vi "Merge_Files.vi"(8 "error in (no error)":errorcluster, 10 "files":refnum<class "IB_CtrFile.lvclass">[](array[class]), 11 "IB_Source_Container in":refnum<class "IB_Source_Container.lvclass">) -> (0 "error out":errorcluster, 3 "IB_Source_Container out":refnum<class "IB_Source_Container.lvclass">)   [LabVIEW 2020, in "IB_Source_Container.lvclass"]
uses:
  <vilib>/AppBuilder/IB_Classes/Source/Container/IB_Source_Container.lvclass
  <vilib>/AppBuilder/IB_Classes/Source/Container/IB_Source_Container.lvclass/IB_Source_Container.ctl
  <vilib>/AppBuilder/IB_Classes/Source/IB_Source.lvclass
  <vilib>/AppBuilder/IB_Classes/Source/File/IB_Source_File.lvclass
  <vilib>/AppBuilder/IB_Classes/Source/File/CtrFile/IB_CtrFile.lvclass
  e:/builds/penguin/labview/branches/2020/dev/dist/vi.lib/AppBuilder/IB_Classes/Source/File/IB_Source_File.lvclass
  e:/builds/penguin/labview/branches/2020/dev/dist/vi.lib/AppBuilder/IB_Classes/Source/IB_Source.lvclass
  e:/builds/penguin/labview/branches/2020/dev/dist/vi.lib/AppBuilder/IB_Classes/Source/File/CtrFile/IB_CtrFile.lvclass
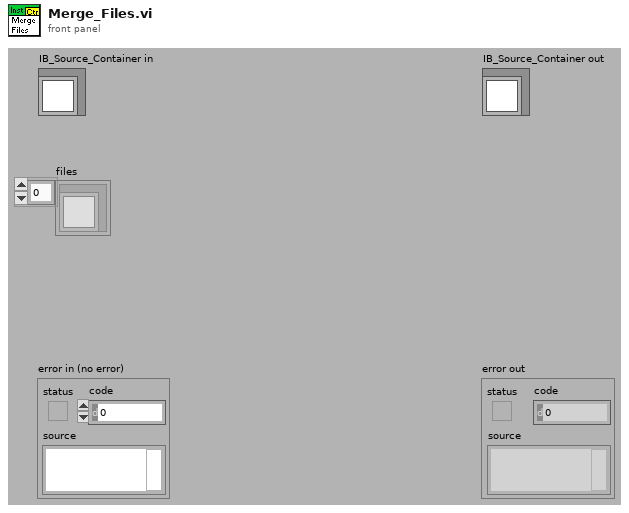
[diagram p1: front panel]
types:
  T1 = typedef "IB_Source.ctl" = cluster{"name":string, "sourceTag":string, "destTag":string, "path":path, "eng_installPath":string, "UI_inBuild?":bool, "str ref?":bool}
  T2 = typedef "IB_Source_File.ctl" = cluster{"Attributes":i16, "RegCOM":bool, "unlock":bool, "shortcuts":refnum<class "IB_Shortcut.lvclass">[], "EXE_install":bool, "CmdArg_install":string, "EXE_uninstall":bool, "CmdArg_uninstall":string}
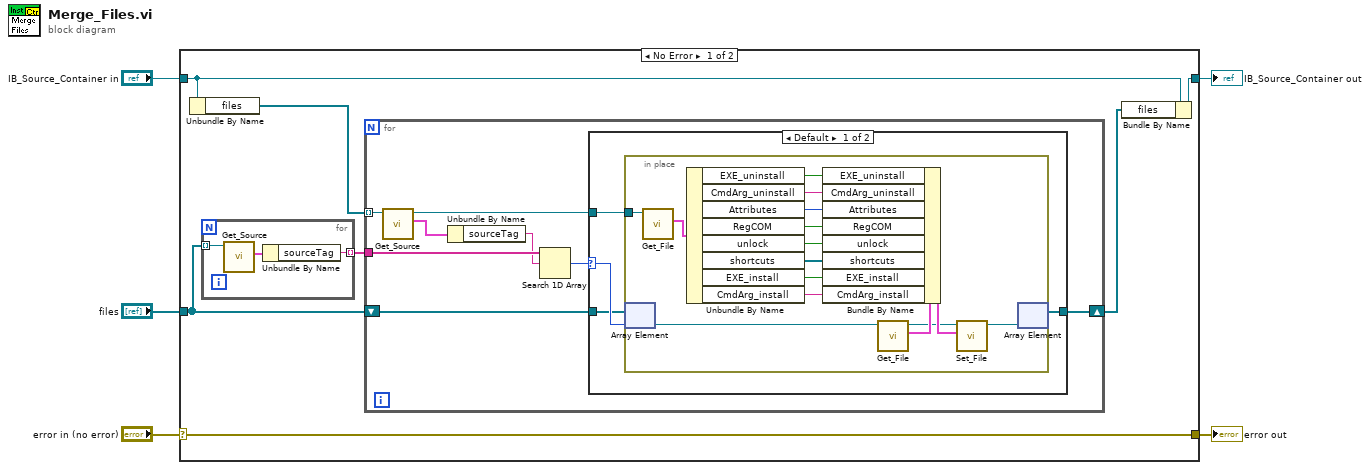
[diagram p0: block diagram]
diagram:
  n1 = case shown="No Error" "error in (no error)" {
    selector: "error in (no error)" -> [w12 w45]
    tunnel: [w12 w45] -> w4
    tunnel: [w9 w44] -> w2
    tunnel: "IB_Source_Container in" -> [w10 w44]
    tunnel: "files" -> [w7 _]
    frame No Error {
      n2 = Unbundle By Name(w10) -> ("files"=w11:refnum<class "IB_CtrFile.lvclass">[])
      n3 = for {
        tunnel: w7 -> [w15] mode=indexing
        tunnel: [w13] -> w6 mode=indexing
        n4 = call <vilib>:"Get_Source.vi"("IB_Source in"=w15) -> ("data"=w14:T1)  [unwired: 1 in, 9 out]
        n5 = Unbundle By Name(w14) -> ("sourceTag"=w13:string)
      }
      n6 = for {
        tunnel: w11 -> [w22] mode=indexing
        tunnel: w6 -> [w21]
        shift-right: [w18] -> w8
        shift-left: w7 -> [w19]
        n7 = call <vilib>:"Get_Source.vi"("IB_Source in"=w22) -> ("data"=w23:T1, "IB_Source out"=w17:refnum<class "IB_CtrFile.lvclass">)  [unwired: 1 in, 8 out]
        n8 = Unbundle By Name(w23) -> ("sourceTag"=w20:string)
        n9 = Search 1D Array(1D array=w21, element=w20) -> (index of element=w16:i32)  [unwired: 1 out]
        n10 = case shown="Default" w16 {
          selector: w16 -> [w27 _]
          tunnel: w17 -> [w24 _]
          tunnel: w19 -> [w26 w43]
          tunnel: [w25 w43] -> w18
          frame Default {
            n11 = in-place {
              in-place-border: w24 -> [w38]
              n12 = in-place-array #1(w26, w27) -> (w40:refnum<class "IB_CtrFile.lvclass">)
              n13 = call <vilib>:"Get_File.vi"("IB_Source_File in"=w38) -> ("data"=w37:T2)  [unwired: 1 in, 9 out]
              n14 = Unbundle By Name(w37) -> ("EXE_uninstall"=w29:bool, "CmdArg_uninstall"=w28:string, "Attributes"=w36:i16, "RegCOM"=w35:bool, "unlock"=w34:bool, "shortcuts"=w33:refnum<class "IB_Shortcut.lvclass">[], "EXE_install"=w31:bool, "CmdArg_install"=w30:string)
              n15 = call <vilib>:"Get_File.vi"("IB_Source_File in"=w40) -> ("data"=w42:T2, "IB_Source_File out"=w39:refnum<class "IB_CtrFile.lvclass">)  [unwired: 1 in, 8 out]
              n16 = Bundle By Name(cluster=w42, "EXE_uninstall"=w29, "CmdArg_uninstall"=w28, "Attributes"=w36, "RegCOM"=w35, "unlock"=w34, "shortcuts"=w33, "EXE_install"=w31, "CmdArg_install"=w30) -> (w41:T2)
              n17 = call <vilib>:"Set_File.vi"("data"=w41, "IB_Source_File in"=w39) -> ("IB_Source_File out"=w32:refnum<class "IB_CtrFile.lvclass">)  [unwired: 1 in, 8 out]
              n18 = in-place-array #1(w32) -> (w25:refnum<class "IB_CtrFile.lvclass">[])  [unwired: 1 out]
            }
          }
          frame -1 {
          }
        }
      }
      n19 = Bundle By Name(cluster=w10, "files"=w8) -> (w9:refnum<class "IB_Source_Container.lvclass">)
    }
    frame Error {
    }
  }
  "error out" <- w4
  "IB_Source_Container out" <- w2
